vi "Const Variable to Save.vi"() -> (4 "shared variable refnum out":refnum<k21>[](array[refnum]))   [LabVIEW 2019]
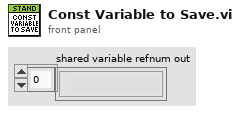
[diagram p1: front panel]
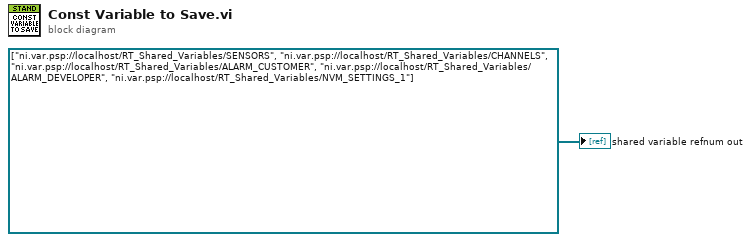
[diagram p0: block diagram]
diagram:
  "shared variable refnum out" <- refnum<k21>[] ["ni.var.psp://localhost/RT_Shared_Variables/SENSORS", "ni.var.psp://localhost/RT_Shared_Variables/CHANNELS", "ni.var.psp://localhost/RT_Shared_Variables/ALARM_CUSTOMER", "ni.var.psp://localhost/RT_Shared_Variables/ALARM_DEVELOPER", "ni.var.psp://localhost/RT_Shared_Variables/NVM_SETTINGS_1"] ("shared variable refnum in")
